vi "Close.vi"(8 "error in (no error)":errorcluster, 11 "Measurement in":refnum<class "Measurement.lvclass">) -> (0 "error out":errorcluster, 3 "Measurement out":refnum<class "Measurement.lvclass">)   [LabVIEW 2017, in "Measurement Actor.lvlib" / "Measurement.lvclass"]
uses:
  Measurement.lvclass
  C:/Program Files (x86)/National Instruments/LabVIEW 2017/vi.lib/ActorFramework/Actor/Actor.lvclass
  Measurement.lvclass/Measurement.ctl
  <vilib>/ActorFramework/Actor/Actor.lvclass/Actor.ctl
  <vilib>/ActorFramework/Message Enqueuer/Message Enqueuer.lvclass/Message Enqueuer.ctl
  <vilib>/ActorFramework/Message Enqueuer/Init from Existing Queue.vi
  <vilib>/ActorFramework/Message Enqueuer/Enqueue.vi
  <vilib>/ActorFramework/Stop Msg/Stop Msg.lvclass
  C:/Program Files (x86)/National Instruments/LabVIEW 2017/vi.lib/ActorFramework/Message/Message.lvclass
  <vilib>/ActorFramework/Message Priority Queue/Priority Enqueue.vi
  Results/Results.lvclass
  <vilib>/ActorFramework/Message Enqueuer/Message Enqueuer.lvclass
  Controller/Messages/Send Results Object/Send Results Object.lvclass
  <vilib>/ActorFramework/Actor/Actor.lvclass
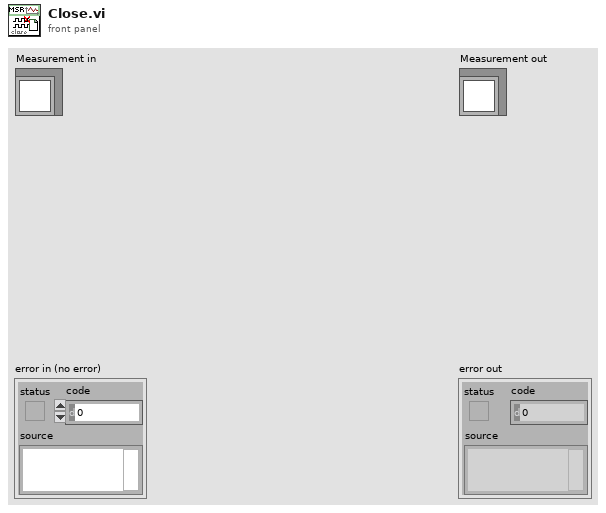
[diagram p1: front panel]
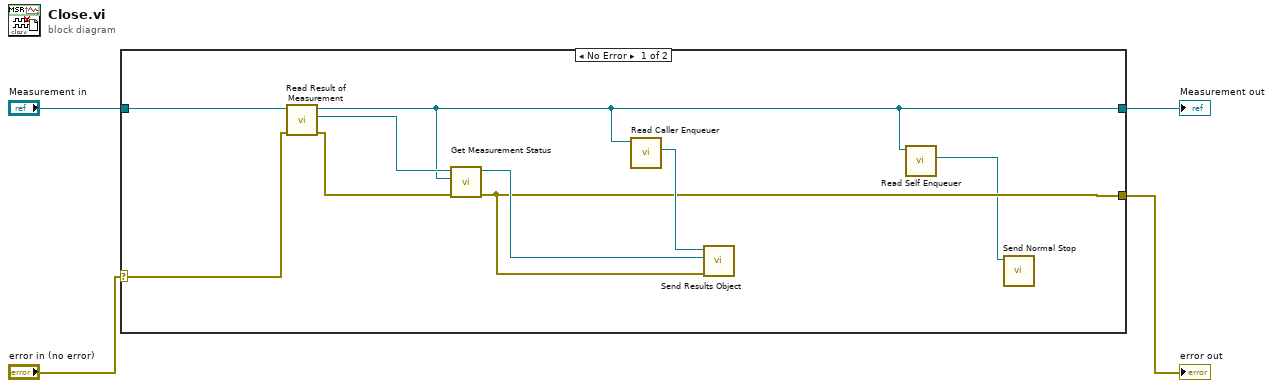
[diagram p0: block diagram]
diagram:
  n1 = case shown="No Error" "error in (no error)" {
    selector: "error in (no error)" -> [w9 w15]
    tunnel: [w7 w15] -> w2
    tunnel: [w6 w14] -> w3
    tunnel: "Measurement in" -> [w11 w14]
    frame No Error {
      n2 = call "Read Result of Measurement.vi"("error in (no error)"=w9, "Measurement in"=w11) -> ("error out"=w8:errorcluster, "Result Actor.lvlib:Results.lvclass"=w10:refnum<class "Results.lvclass">, "Measurement out"=w6:refnum<class "Measurement.lvclass">)  [unwired: 7 in]
      n3 = call-dynamic "Get Measurement Status.vi"("error in (no error)"=w8, "Measurement.lvclass"=w6, "Results in"=w10) -> ("error out"=w7:errorcluster, "Results out"=w13:refnum<class "Results.lvclass">)  [unwired: 7 in]
      n4 = call <vilib>:"Read Caller Enqueuer.vi"("Actor"=w6) -> ("Caller Enqueuer"=w12:refnum<class "Message Enqueuer.lvclass">)  [unwired: 10 in]
      n5 = call "Send Results Object.vi"("error in (no error)"=w7, "Results.lvclass"=w13, "Message Enqueuer in"=w12) -> ()  [unwired: 7 in, 2 out]
      n6 = call <vilib>:"Read Self Enqueuer.vi"("Actor"=w6) -> ("Self Enqueuer"=w5:refnum<class "Message Enqueuer.lvclass">)  [unwired: 10 in]
      n7 = call <vilib>:"Send Normal Stop.vi"("Message Enqueuer"=w5) -> ()  [unwired: 10 in, 1 out]
    }
    frame Error {
    }
  }
  "error out" <- w2
  "Measurement out" <- w3
